vi "main_wash.vi"(4 "Stop":refnum<vi>, 5 "Main wash state":T1, 6 "timer":refnum<vi>, 7 "Vehicle out of position":refnum<vi>, 8 "Clear water rinse":refnum<vi>, 9 "Main high pressure wash":refnum<vi>, 10 "Soap application":refnum<vi>, 11 "Cycle Switch":refnum<vi>) -> ()   [LabVIEW 2024]
uses:
  main_wash_state.ctl
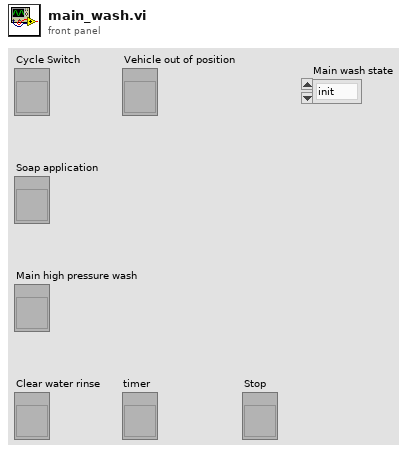
[diagram p1: front panel]
types:
  T1 = typedef "main_wash_state.ctl" = enum16{"init", "soap application", "main high pressure wash", "clear water rinse", "end"}
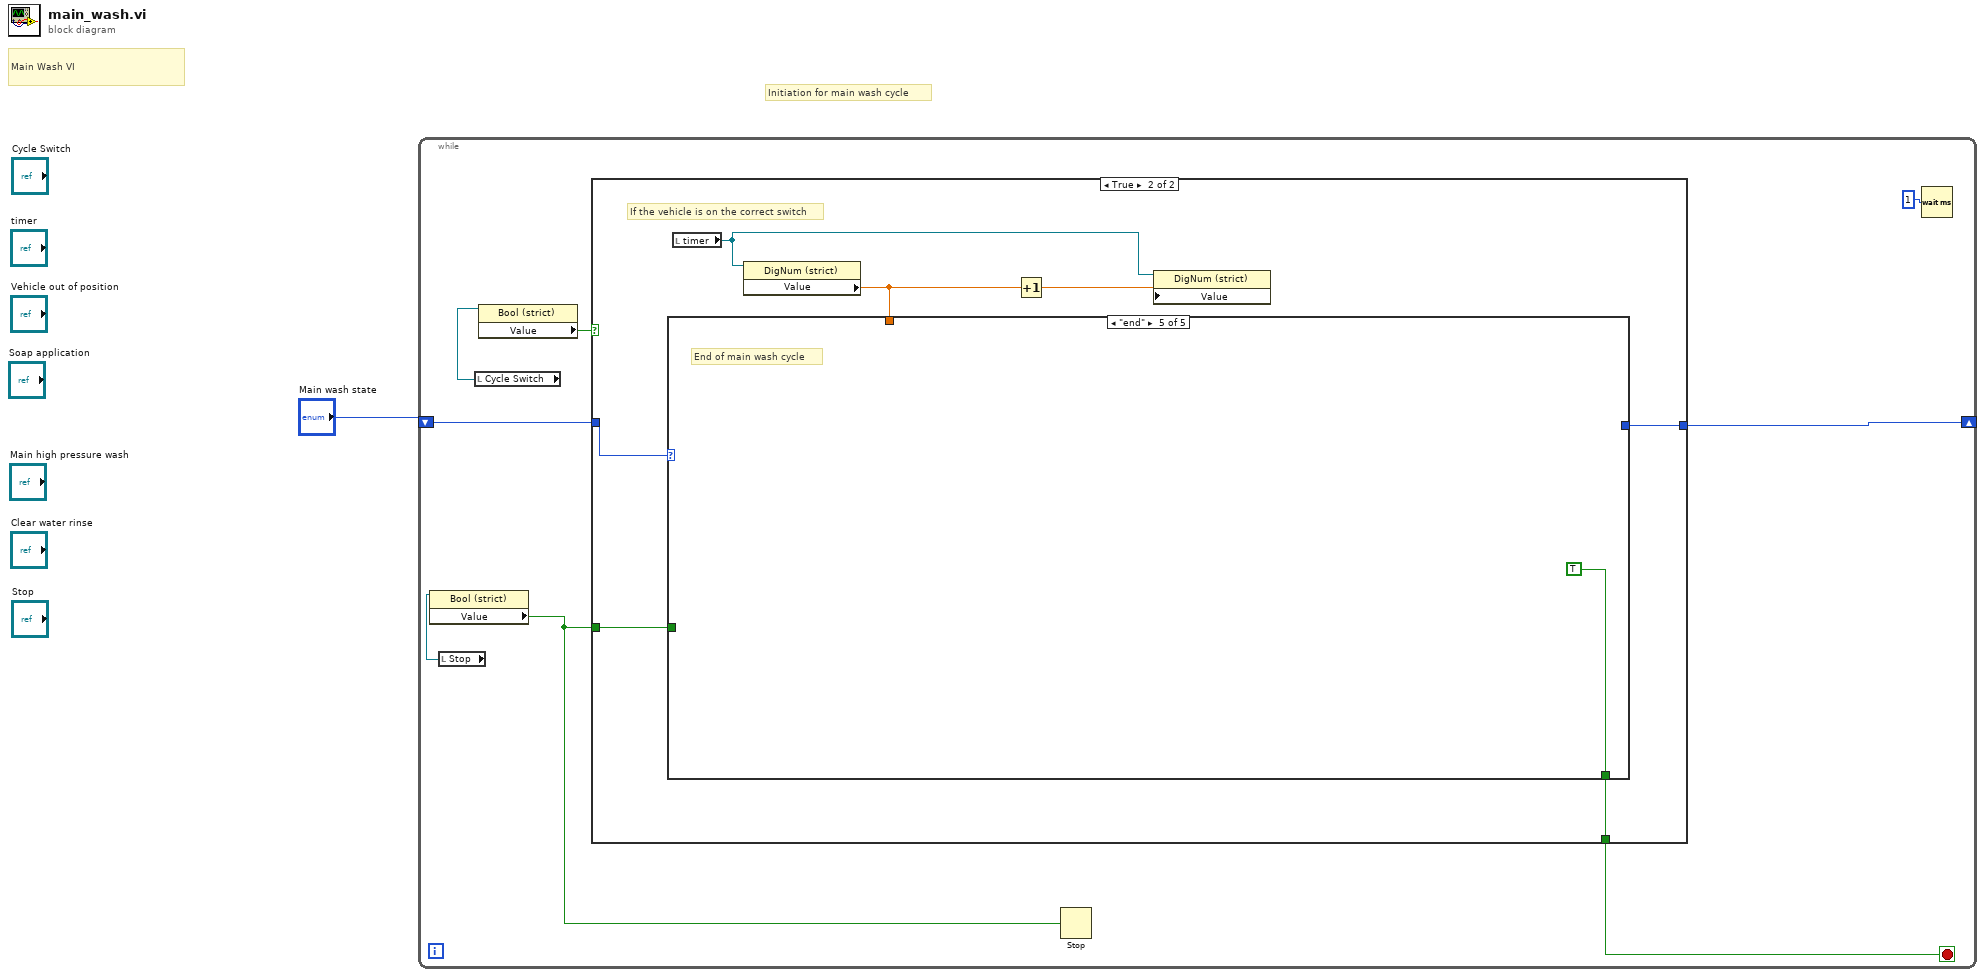
[diagram p0: block diagram]
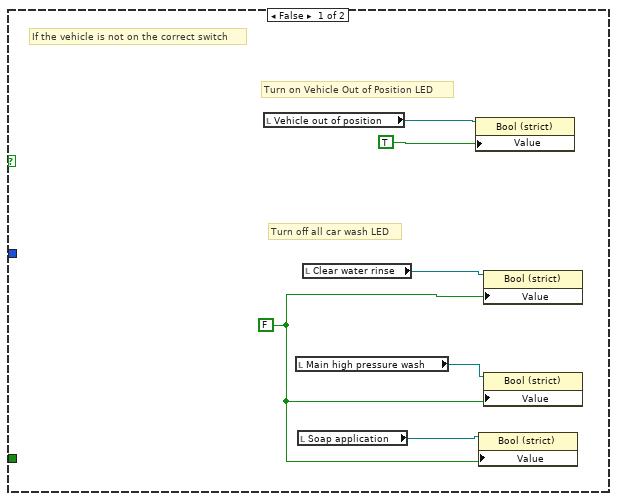
[diagram p2: hidden frame]
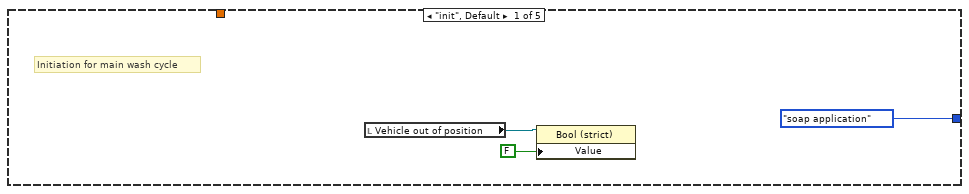
[diagram p3: hidden frame]
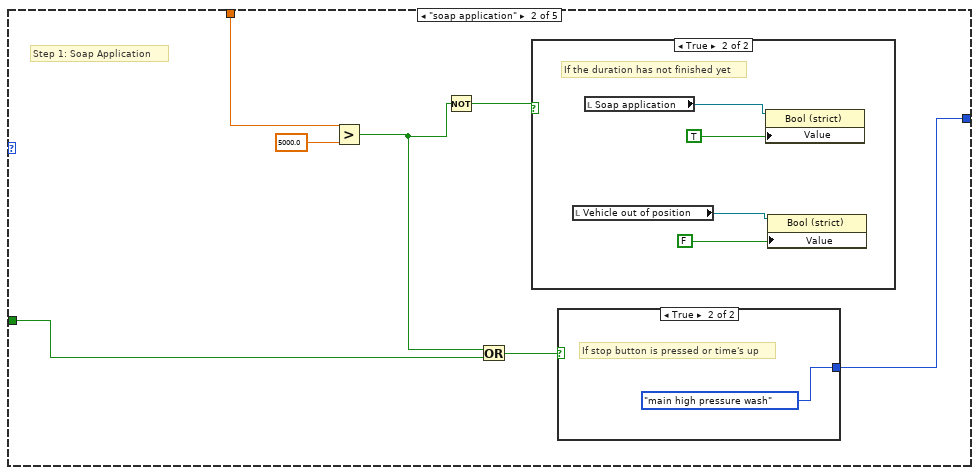
[diagram p4: hidden frame]
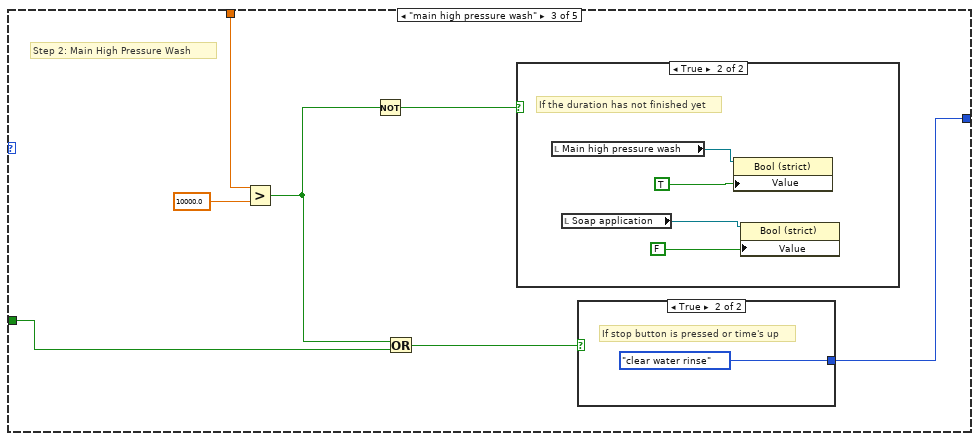
[diagram p7: hidden frame]
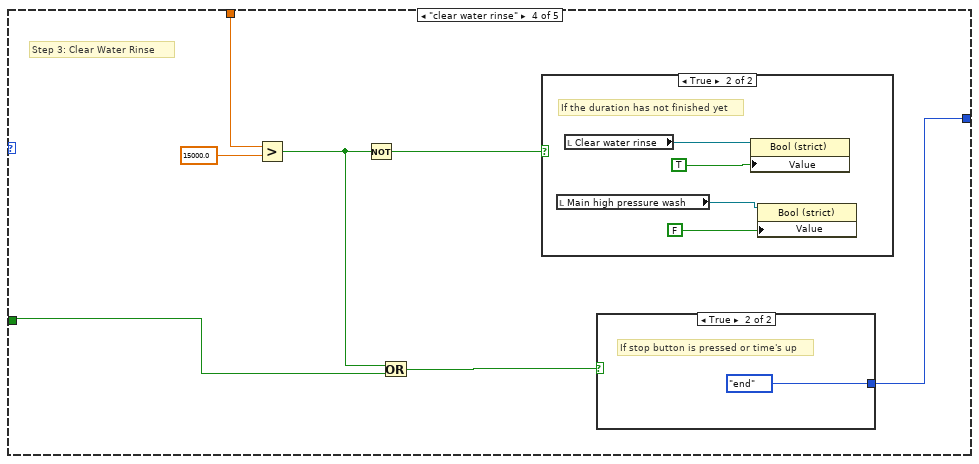
[diagram p10: hidden frame]
diagram:
  # "Initiation for main wash cycle"
  # "Main Wash VI"
  n1 = while {
    shift-right: [w3] -> _
    shift-left: "Main wash state" -> [w2]
    stop <- w6 stop-if-true
    n2 = local read "Stop"() -> (w5:refnum<vi>)
    n3 = property class="Bool (strict)"(reference=w5) -> ("Value"=w8:bool)  [unwired: 1 in, 2 out]
    n4 = local read "Cycle Switch"() -> (w4:refnum<vi>)
    n5 = property class="Bool (strict)"(reference=w4) -> ("Value"=w7:bool)  [unwired: 1 in, 2 out]
    n6 = case shown="True" w7 {
      tunnel: [_ w22] -> w3
      tunnel: [_ w19] -> w6
      tunnel: w8 -> [_ w16]
      tunnel: w2 -> [_ w18]
      frame False {
        w14 = FALSE ("Under Body Wash")
        # "Turn off all car wash LED"
        # "Turn on Vehicle Out of Position LED"
        # "If the vehicle is not on the correct switch"
        n7 = local read "Vehicle out of position"() -> (w13:refnum<vi>)
        n8 = local read "Main high pressure wash"() -> (w11:refnum<vi>)
        n9 = local read "Soap application"() -> (w10:refnum<vi>)
        n10 = local read "Clear water rinse"() -> (w12:refnum<vi>)
        n11 = property class="Bool (strict)"(reference=w13, "Value"=TRUE ("Under Body Wash")) -> ()  [unwired: 1 in, 2 out]
        n12 = property class="Bool (strict)"(reference=w10, "Value"=w14) -> ()  [unwired: 1 in, 2 out]
        n13 = property class="Bool (strict)"(reference=w12, "Value"=w14) -> ()  [unwired: 1 in, 2 out]
        n14 = property class="Bool (strict)"(reference=w11, "Value"=w14) -> ()  [unwired: 1 in, 2 out]
      }
      frame True {
        # "If the vehicle is on the correct switch"
        n15 = local read "timer"() -> (w17:refnum<vi>)
        n16 = property class="DigNum (strict)"(reference=w17) -> ("Value"=w20:dbl)  [unwired: 1 in, 2 out]
        n17 = case shown="\"end\"" w18 {
          tunnel: [main_wash_state."soap application" w28 w40 w52 _] -> w22
          tunnel: w20 -> [_ w32 w41 w53 _]
          tunnel: [_ _ _ _ TRUE] -> w19
          tunnel: w16 -> [_ w26 w38 w50 _]
          frame "init", Default {
            # "Initiation for main wash cycle"
            n18 = local read "Vehicle out of position"() -> (w23:refnum<vi>)
            n19 = property class="Bool (strict)"(reference=w23, "Value"=FALSE ("Under Body Wash")) -> ()  [unwired: 1 in, 2 out]
          }
          frame "soap application" {
            # "Step 1: Soap Application"
            n20 = Greater?(x=w32, y=5000.0) -> (0:w30:bool)
            n21 = Not(x=w30) -> (.not. x?=w31:bool)
            n22 = Or(x=w30, y=w26) -> (x .or. y?=w29:bool)
            n23 = case shown="True" w31 {
              frame False {
              }
              frame True {
                # "If the duration has not finished yet"
                n24 = local read "Vehicle out of position"() -> (w35:refnum<vi>)
                n25 = local read "Soap application"() -> (w36:refnum<vi>)
                n26 = property class="Bool (strict)"(reference=w36, "Value"=TRUE ("Under Body Wash")) -> ()  [unwired: 1 in, 2 out]
                n27 = property class="Bool (strict)"(reference=w35, "Value"=FALSE ("Under Body Wash")) -> ()  [unwired: 1 in, 2 out]
              }
            }
            n28 = case shown="True" w29 {
              tunnel: [_ main_wash_state."main high pressure wash"] -> w28
              frame False {
              }
              frame True {
                # "If stop button is pressed or time's up"
              }
            }
          }
          frame "main high pressure wash" {
            # "Step 2: Main High Pressure Wash"
            n29 = Greater?(x=w41, y=10000.0) -> (0:w43:bool)
            n30 = Not(x=w43) -> (.not. x?=w44:bool)
            n31 = Or(x=w43, y=w38) -> (x .or. y?=w42:bool)
            n32 = case shown="True" w44 {
              frame False {
              }
              frame True {
                # "If the duration has not finished yet"
                n33 = local read "Main high pressure wash"() -> (w46:refnum<vi>)
                n34 = local read "Soap application"() -> (w45:refnum<vi>)
                n35 = property class="Bool (strict)"(reference=w46, "Value"=TRUE ("Under Body Wash")) -> ()  [unwired: 1 in, 2 out]
                n36 = property class="Bool (strict)"(reference=w45, "Value"=FALSE ("Under Body Wash")) -> ()  [unwired: 1 in, 2 out]
              }
            }
            n37 = case shown="True" w42 {
              tunnel: [_ main_wash_state."clear water rinse"] -> w40
              frame False {
              }
              frame True {
                # "If stop button is pressed or time's up"
              }
            }
          }
          frame "clear water rinse" {
            # "Step 3: Clear Water Rinse"
            n38 = Greater?(x=w53, y=15000.0) -> (0:w55:bool)
            n39 = Not(x=w55) -> (.not. x?=w56:bool)
            n40 = Or(x=w55, y=w50) -> (x .or. y?=w54:bool)
            n41 = case shown="True" w56 {
              frame False {
              }
              frame True {
                # "If the duration has not finished yet"
                n42 = local read "Main high pressure wash"() -> (w57:refnum<vi>)
                n43 = local read "Clear water rinse"() -> (w58:refnum<vi>)
                n44 = property class="Bool (strict)"(reference=w58, "Value"=TRUE ("Under Body Wash")) -> ()  [unwired: 1 in, 2 out]
                n45 = property class="Bool (strict)"(reference=w57, "Value"=FALSE ("Under Body Wash")) -> ()  [unwired: 1 in, 2 out]
              }
            }
            n46 = case shown="True" w54 {
              tunnel: [_ main_wash_state."end"] -> w52
              frame False {
              }
              frame True {
                # "If stop button is pressed or time's up"
              }
            }
          }
          frame "end" {
            # "End of main wash cycle"
          }
        }
        n47 = Increment(x=w20) -> (x+1=w21:dbl)
        n48 = property class="DigNum (strict)"(reference=w17, "Value"=w21) -> ()  [unwired: 1 in, 2 out]
      }
    }
    n49 = Stop(stop? (T)=w8) -> ()
    n50 = Wait (ms)(milliseconds to wait=u32 1) -> ()  [unwired: 1 out]
  }
